vi "TCP read variant.vi"(0 "connection ID":refnum<k5>, 9 "timeout ms (25000)":i32=5000, 11 "error in (no error)":errorcluster) -> (4 "connection ID out":refnum<k5>, 6 "bytes read":i32, 8 "data out":string, 15 "error out":errorcluster)   [LabVIEW 2015]
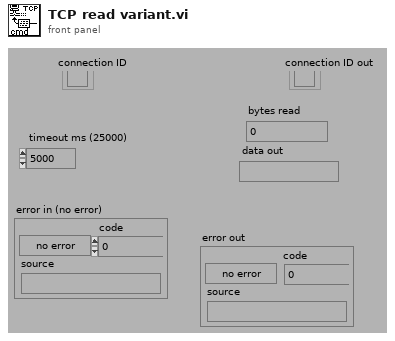
[diagram p1: front panel]
types:
  T1 = enum16{"Standard", "Buffered", "CRLF", "Immediate"}
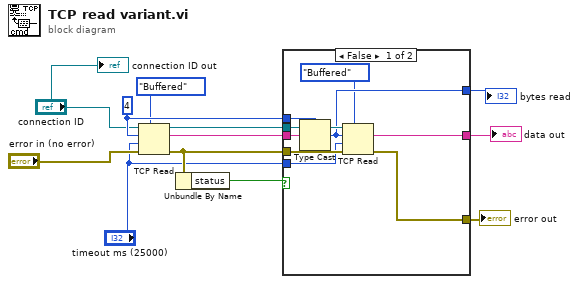
[diagram p0: block diagram]
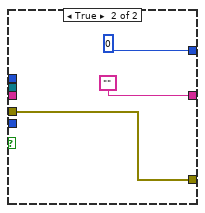
[diagram p2: hidden frame]
diagram:
  w12 = 4
  n1 = TCP Read(connection ID="connection ID", bytes to read=w12, error in (no error)="error in (no error)", 7:T1."Buffered" ("mode (standard)"), 9:"timeout ms (25000)") -> (connection ID out=w10:refnum<k5>, data out=w11:string, error out=w7:errorcluster)
  n2 = Unbundle By Name(w7) -> ("status"=w6:bool)
  n3 = case shown="False" w6 {
    tunnel: w7 -> [w21 w24]
    tunnel: "timeout ms (25000)" -> [w20 _]
    tunnel: w10 -> [w19 _]
    tunnel: w11 -> [w18 _]
    tunnel: w12 -> [w17 _]
    tunnel: [w16 w24] -> w5
    tunnel: [w15 ""] -> w4
    tunnel: [w14 0] -> w3
    frame False {
      n4 = Type Cast(type=w17, x=w18) -> (*(type *) &x=w14:i32)
      n5 = TCP Read(connection ID=w19, bytes to read=w14, error in (no error)=w21, 7:T1."Buffered" ("mode (standard)"), 9:w20) -> (data out=w15:string, error out=w16:errorcluster)  [unwired: 1 out]
    }
    frame True {
    }
  }
  "error out" <- w5
  "data out" <- w4
  "bytes read" <- w3
  "connection ID out" <- "connection ID"
